vi "Untitled 2.vi"() -> ()   [LabVIEW 2016]
uses:
  System.Net.Http
panel:
  out "ToString":string
  out "AuthorizationHeader":string
  in  "password":string="gamma2018"
  in  "Username":string="admin"
  out "string":string
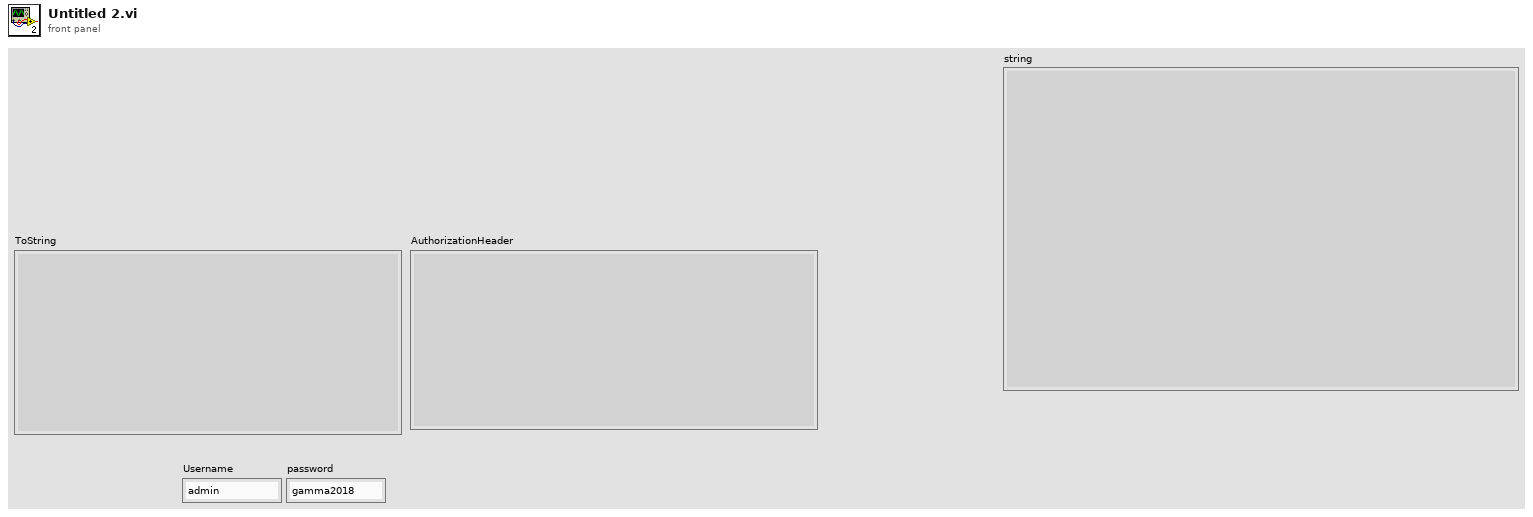
[diagram p1: front panel]
types:
  T1 = cluster{"realm":string, "qop":string, "nounce":string, "opaque":string}
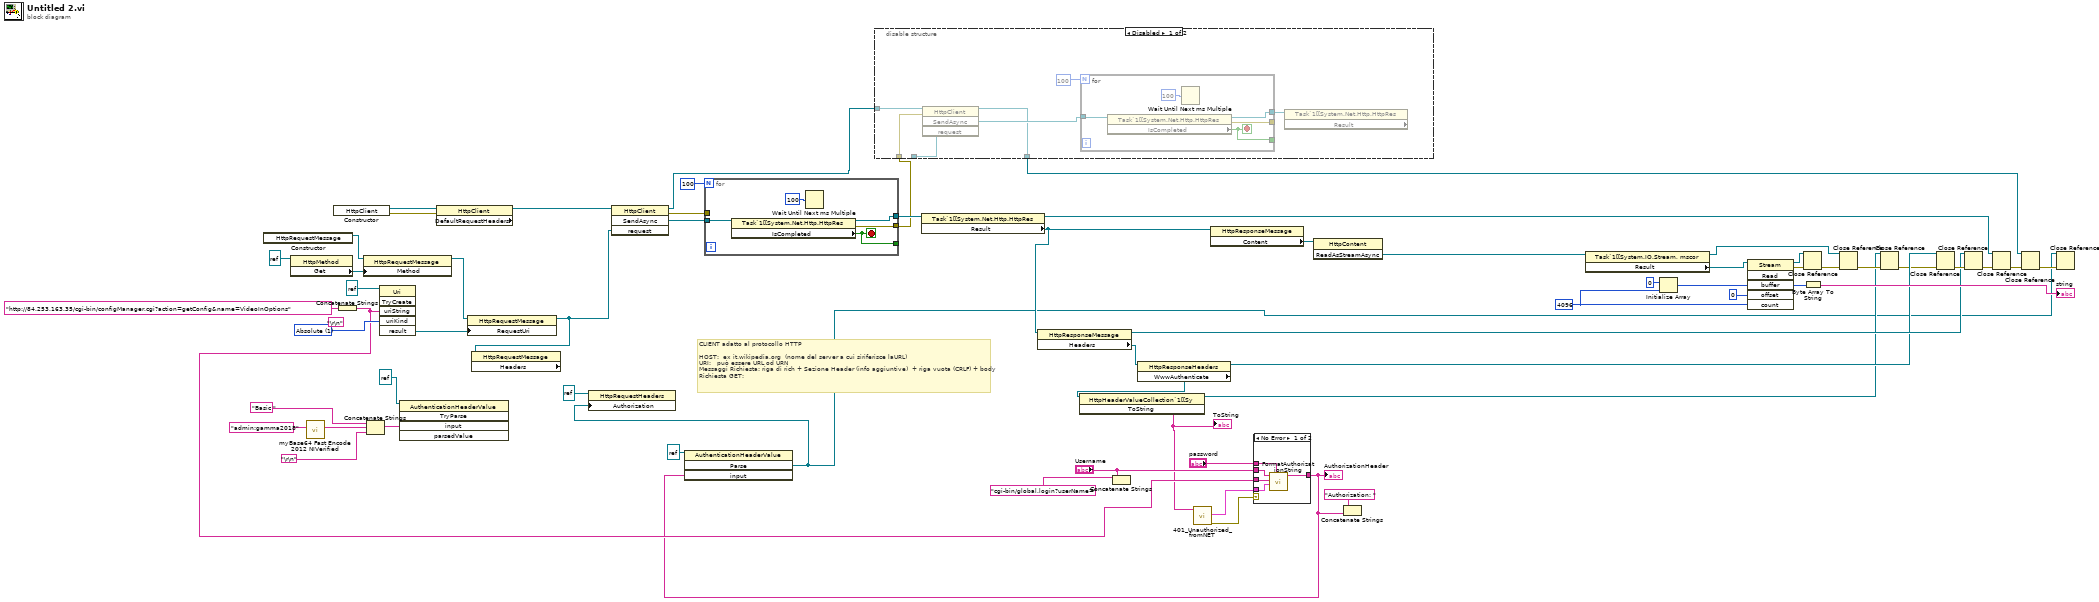
[diagram p0: block diagram]
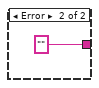
[diagram p2: hidden frame]
diagram:
  (unwired) "\r\n"
  w48 = 4096 ("dimension size")
  w62 = 1 items=["RelativeOrAbsolute", "Absolute", "Relative"] ("uriKind")
  # "CLIENT adatto al protocollo HTTP\n\nHOST:  ex it.wikipedia.org  (nome del server a cui siriferisce laURL)\nURI:   può essere URL od URN\nMessaggi Richiesta: riga di rich + Sezione Header (info aggiuntive)  + riga vuota (CRLF) + body\nRichiesta GET:"
  n1 = constructor class="HttpRequestMessage"() -> (reference out=w59:refnum<k24>)  [unwired: 3 in, 2 out]
  n2 = property class="HttpMethod"(reference=refnum<k24> refnum) -> ("Get"=w58:refnum<k24>)  [unwired: 1 in, 2 out]
  n3 = call "myBase64 Fast Encode 2012 NIVerified.vi"("string in (not encoded)"="admin:gamma2018") -> ("string out (base64-encoded)"=w31:string)  [unwired: 9 in, 1 out]
  n4 = constructor class="HttpClient"() -> (reference out=w35:refnum<k24>, error out=w34:errorcluster)  [unwired: 3 in, 1 out]
  n5 = Concatenate Strings("http://84.253.163.35/cgi-bin/configManager.cgi?action=getConfig&name=VideoInOptions") -> (w17:string)
  n6 = property class="HttpRequestMessage"(reference=w59, "Method"=w58) -> (reference out=w24:refnum<k24>)  [unwired: 1 in, 1 out]
  n7 = Concatenate Strings("Basic ", w31, "\r\n") -> (w23:string)
  n8 = invoke class="Uri" method="TryCreate"(reference=refnum<k24> refnum, "uriString"=w17, "uriKind"=w62) -> ("result"=w25:refnum<k24>)  [unwired: 3 in, 5 out]
  n9 = invoke class="AuthenticationHeaderValue" method="TryParse"(reference=refnum<k24> refnum ("Authorization"), "input"=w23) -> ()  [unwired: 3 in, 5 out]
  n10 = property class="HttpClient" props=["DefaultRequestHeaders"](reference=w35, error in=w34) -> (reference out=w32:refnum<k24>)  [unwired: 2 out]
  n11 = property class="HttpRequestMessage"(reference=w24, "RequestUri"=w25) -> (reference out=w2:refnum<k24>)  [unwired: 1 in, 1 out]
  n12 = property class="HttpRequestMessage" props=["Headers"](reference=w2) -> ()  [unwired: 1 in, 3 out]
  n13 = invoke class="HttpClient" method="SendAsync"(reference=w32, "request"=w2) -> (reference out=w1:refnum<k24>, error out=w7:errorcluster, "SendAsync"=w54:refnum<k24>)  [unwired: 2 in, 1 out]
  n14 = for {
    N: 100 -> [_]
    tunnel: w54 -> [w68]
    tunnel: [w67] -> _
    tunnel: [w65] -> w55
    tunnel: [w64] -> w27
    tunnel: w7 -> [_]
    stop <- w67 stop-if-true
    n15 = property class="Task`1[[System.Net.Http.HttpRes"(reference=w68) -> (reference out=w65:refnum<k24>, error out=w64:errorcluster, "IsCompleted"=w67:bool)  [unwired: 1 in]
    n16 = Wait Until Next ms Multiple(millisecond multiple=u32 100) -> ()  [unwired: 1 out]
  }
  n17 = disable-structure shown="Disabled" {
    disable-tunnel: w27 -> [w75 _]
    disable-tunnel: w1 -> [w71 w81]
    disable-tunnel: [w70 w81] -> w26
    disable-tunnel: _ -> [w69 _]
    frame Disabled {
      n18 = invoke class="HttpClient" method="SendAsync"(reference=w71, error in=w75, "request"=w69) -> (reference out=w70:refnum<k24>, "SendAsync"=w74:refnum<k24>)  [unwired: 1 in, 2 out]
      n19 = for {
        N: 100 -> [_]
        tunnel: w74 -> [w80]
        tunnel: [w79] -> _
        tunnel: [w77] -> w72
        tunnel: [w76] -> _
        stop <- w79 stop-if-true
        n20 = property class="Task`1[[System.Net.Http.HttpRes"(reference=w80) -> (reference out=w77:refnum<k24>, error out=w76:errorcluster, "IsCompleted"=w79:bool)  [unwired: 1 in]
        n21 = Wait Until Next ms Multiple(millisecond multiple=u32 100) -> ()  [unwired: 1 out]
      }
      n22 = property class="Task`1[[System.Net.Http.HttpRes" props=["Result"](reference=w72) -> ()  [unwired: 1 in, 3 out]
    }
    frame Enabled {
    }
  }
  n23 = property class="Task`1[[System.Net.Http.HttpRes"(reference=w55) -> (reference out=w37:refnum<k24>, "Result"=w15:refnum<k24>)  [unwired: 1 in, 1 out]
  n24 = property class="HttpResponseMessage"(reference=w15) -> (reference out=w38:refnum<k24>, "Headers"=w14:refnum<k24>)  [unwired: 1 in, 1 out]
  n25 = Concatenate Strings("cgi-bin/global.login?userName=", "Username") -> ()  [unwired: 1 out]
  n26 = property class="HttpResponseHeaders"(reference=w14) -> (reference out=w13:refnum<k24>, "WwwAuthenticate"=w10:refnum<k24>)  [unwired: 1 in, 1 out]
  n27 = invoke class="HttpHeaderValueCollection`1[[Sy" method="ToString"(reference=w10) -> (reference out=w9:refnum<k24>, "ToString"=w8:string)  [unwired: 2 in, 1 out]
  "ToString" <- w8
  n28 = call "401_Unauthorized_fromNET.vi"("headers"=w8) -> ("error out"=w16:errorcluster, "ServerInfo"=w22:T1)  [unwired: 9 in]
  n29 = property class="HttpResponseMessage"(reference=w15) -> ("Content"=w53:refnum<k24>)  [unwired: 1 in, 2 out]
  n30 = case shown="No Error" w16 {
    tunnel: w22 -> [w86 _]
    tunnel: "Username" -> [w85 _]
    tunnel: w17 -> [w83 _]
    tunnel: "password" -> [w84 _]
    tunnel: [w82 ""] -> w6
    frame No Error {
      n31 = call "FormatAuthorizationString.vi"("password"=w84, "ServerInfo"=w86, "String in"=w83, "Username"=w85) -> ("String out"=w82:string)  [unwired: 7 in]
    }
    frame Error {
    }
  }
  "AuthorizationHeader" <- w6
  n32 = invoke class="AuthenticationHeaderValue" method="Parse"(reference=refnum<k24> refnum, "input"=w6) -> ("Parse"=w4:refnum<k24>)  [unwired: 2 in, 3 out]
  n33 = property class="HttpRequestHeaders"(reference=refnum<k24> refnum ("Headers"), "Authorization"=w4) -> ()  [unwired: 1 in, 2 out]
  n34 = invoke class="HttpContent" method="ReadAsStreamAsync"(reference=w53) -> ("ReadAsStreamAsync"=w52:refnum<k24>)  [unwired: 2 in, 2 out]
  n35 = Concatenate Strings("Authorization: " ("string"), w6) -> ()  [unwired: 1 out]
  n36 = property class="Task`1[[System.IO.Stream, mscor"(reference=w52) -> (reference out=w42:refnum<k24>, "Result"=w45:refnum<k24>)  [unwired: 1 in, 1 out]
  n37 = Initialize Array(u8 0, w48) -> (w50:u8[])
  n38 = invoke class="Stream" method="Read"(reference=w45, "buffer"=w50, "offset"=0, "count"=w48) -> (reference out=w43:refnum<k24>, error out=w44:errorcluster, "buffer"=w47:u8[])  [unwired: 2 in, 3 out]
  n39 = Close Reference(reference=w43, error in (no error)=w44) -> (error out=w63:errorcluster)
  n40 = Byte Array To String(unsigned byte array=w47) -> (string=→"string":string)
  n41 = Close Reference(reference=w42, error in (no error)=w63) -> (error out=w12:errorcluster)
  n42 = Close Reference(reference=w9, error in (no error)=w12) -> (error out=w11:errorcluster)
  n43 = Close Reference(reference=w13, error in (no error)=w11) -> (error out=w39:errorcluster)
  n44 = Close Reference(reference=w38, error in (no error)=w39) -> (error out=w41:errorcluster)
  n45 = Close Reference(reference=w37, error in (no error)=w41) -> (error out=w40:errorcluster)
  n46 = Close Reference(reference=w26, error in (no error)=w40) -> (error out=w36:errorcluster)
  n47 = Close Reference(reference=w4, error in (no error)=w36) -> ()  [unwired: 1 out]
